vi "Framework Test.vi"() -> ()   [LabVIEW 2017]
uses:
  Typedefs/DSF Engine Framework Configuration.ctl
  Typedefs/DSF Engine Plugin Configuration.ctl
  Typedefs/DSF Timing Info.ctl
  Typedefs/DSF Engine Plugin Thread Configuration.ctl
  Typedefs/DSF Settings Info.ctl
  Typedefs/DSF Engine Transfer Group Configuration.ctl
  Typedefs/DSF Direction.ctl
  Typedefs/DSF Engine Transfer Configuration.ctl
  Typedefs/DSF Byte Order.ctl
  Typedefs/DSF Engine Channel Configuration.ctl
  Typedefs/DSF Data Type.ctl
  Typedefs/DSF Timeout Behavior.ctl
  Classes/Framework/Framework Options.ctl
  Typedefs/DSF FIFO Options.ctl
  Classes/Thread/Thread Options.ctl
  Typedefs/DSF Plugin Options.ctl
  Typedefs/DSF Performance Options.ctl
  Classes/Framework/Data Server Options.ctl
  <vilib>/NI/Memory Manager/Classes/Pointer/Pointer.lvclass/Pointer.ctl
  <vilib>/NI/Memory Manager/Classes/Pointer/Write Bool.vi
  <vilib>/NI/Memory Manager/Classes/Pointer/Write DBL.vi
  <vilib>/NI/Memory Manager/Classes/Pointer/Read Bool.vi
  <vilib>/NI/Memory Manager/Classes/Pointer/Set Address.vi
  <vilib>/NI/Memory Manager/Classes/Pointer/Set Size.vi
  <vilib>/NI/Memory Manager/Classes/Pointer/Set Internal.vi
  <vilib>/NI/Memory Manager/Classes/Pointer/Write (No Check).vi
  <vilib>/NI/Memory Manager/Classes/Pointer/Write (No Check) Bool.vi
  <vilib>/NI/Memory Manager/Classes/Pointer/Check Move.vi
  <vilib>/NI/Memory Manager/Classes/Pointer/Check Null Pointer.vi
  <vilib>/NI/Memory Manager/Classes/Pointer/Clear (No Check).vi
  <vilib>/NI/Memory Manager/Classes/Pointer/Check Length.vi
  <vilib>/NI/Memory Manager/Classes/Pointer/Write (No Check) DBL.vi
  <vilib>/NI/Memory Manager/Classes/Pointer/Read (No Check).vi
  <vilib>/NI/Memory Manager/Classes/Pointer/Read (No Check) Bool.vi
  <vilib>/NI/Memory Manager/Classes/Pointer/Get Internal.vi
  <vilib>/NI/Memory Manager/Classes/Pointer/Errors.vi
  <vilib>/NI/Memory Manager/Classes/Pointer/Zone.vi
  <vilib>/NI/Memory Manager/Classes/Pointer/Check Count.vi
  <vilib>/NI/Memory Manager/Classes/Pointer/Check Bounds (Power of 2).vi
  <vilib>/NI/Memory Manager/Classes/Pointer/Null Pointer.vi
  <vilib>/NI/Memory Manager/Classes/Pointer/Is Null.vi
  <vilib>/NI/Memory Manager/Classes/Pointer/Check Bounds (Pointer).vi
  <vilib>/NI/Memory Manager/Classes/Pointer/Create Error.vi
  <vilib>/NI/Memory Manager/Classes/Pointer/Out of Bounds.vi
  <vilib>/NI/Memory Manager/Classes/Pointer/Check Bounds.vi
  <vilib>/NI/Memory Manager/Constants/Constants.vi
  <vilib>/NI/Memory Manager/Constants/Library Name.vi
  <vilib>/NI/Memory Manager/Classes/Pointer/Pointer Error Info.vi
  <vilib>/NI/Memory Manager/Constants/Pointer Class Name.vi
  <vilib>/NI/Memory Manager/Classes/Pointer/Write Pointer Size to Error.vi
  <vilib>/NI/Memory Manager/Classes/Pointer/Check Bounds (Buffer).vi
  <vilib>/NI/Memory Manager/Classes/Pointer/Buffer Underflow.vi
  <vilib>/NI/Memory Manager/VIs/New Error Cluster.vi
  <vilib>/NI/Memory Manager/VIs/New Error Cluster (512B).vi
  <vilib>/NI/Memory Manager/VIs/Set Error Status.vi
  <vilib>/NI/Memory Manager/VIs/Set Error Code.vi
  <vilib>/NI/Memory Manager/VIs/Set Error Source.vi
  <vilib>/NI/Memory Manager/VIs/Write String to Source.vi
  <vilib>/NI/Memory Manager/VIs/Write Numeric to Source.vi
  <vilib>/NI/Memory Manager/VIs/Write Numeric Scalar to Source (Base10 U64).vi
  Classes/Configuration/Channel Count (Framework).vi
  <vilib>/NI/Memory Manager/Classes/Pointer/Pointer.lvclass
  Classes/Framework/Framework.lvclass
  Classes/Configuration/Configuration Session.lvclass
  DSF Core.lvlib
  Classes/Thread/Thread.lvclass
panel:
  in  "first channel":dbl format="%.3f"
  out "iteration":u64
  out "error out":errorcluster
  in  "framework options":T1={"FIFO Options"={"Infinite Timeouts"=FALSE}, "Thread Options"={"Show FP On Call"=TRUE, "Close FP After Call"=TRUE, "Allow Debugging"=TRUE}, "Plugin Options"={"Default Components"=TRUE}, "Performance Options"={"Measure Period"=TRUE, "Measure Rx/Tx Duration"=TRUE}, "Data Server Options"={"Enable Data Server"=TRUE, "Period"=50}} {"Data Server Options"."Period" format="%d ms"}
  in  "framework configuration":T7
  in  "stop":bool
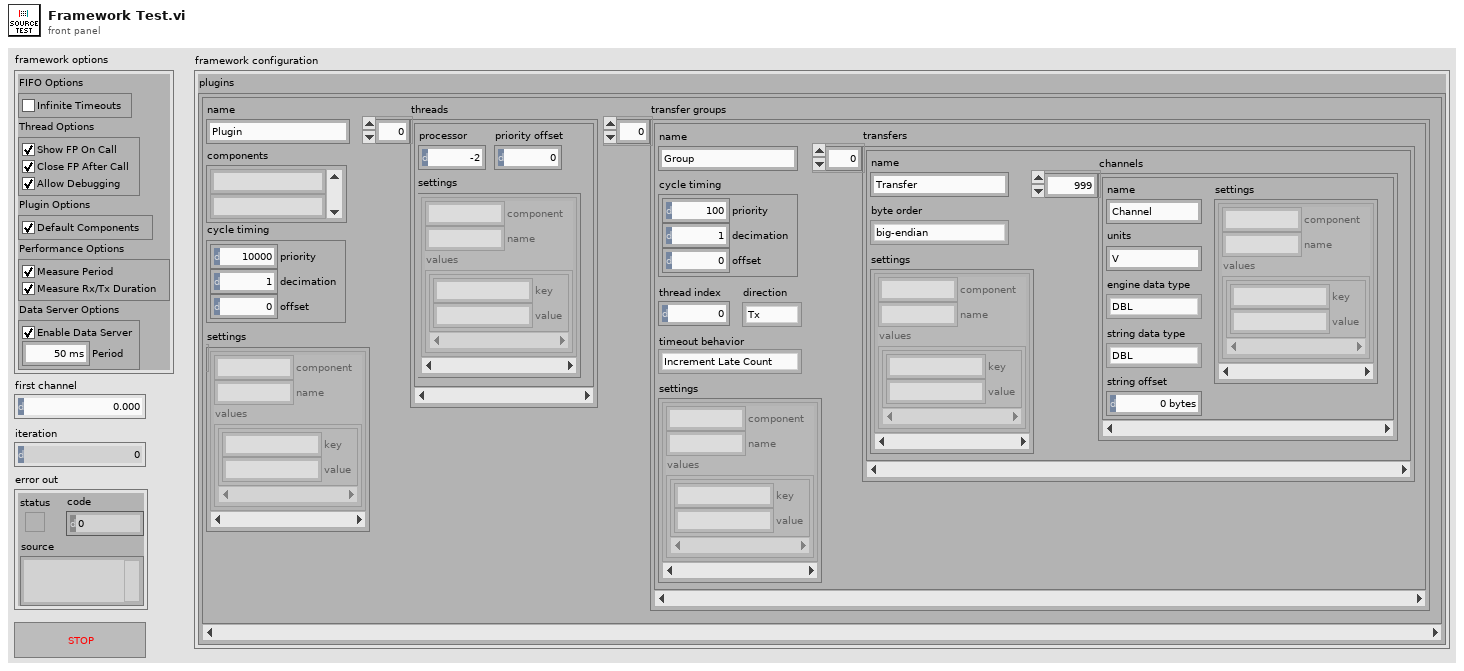
[diagram p1: front panel]
types:
  T1 = typedef "DSF Core.lvlib/Framework.lvclass/Framework Options.ctl" = cluster{"FIFO Options":T2, "Thread Options":T3, "Plugin Options":T4, "Performance Options":T5, "Data Server Options":T6}
  T2 = typedef "DSF Core.lvlib/Framework.lvclass/DSF FIFO Options.ctl" = cluster{"Infinite Timeouts":bool}
  T3 = typedef "DSF Core.lvlib/Thread.lvclass/Thread Options.ctl" = cluster{"Show FP On Call":bool, "Close FP After Call":bool, "Allow Debugging":bool}
  T4 = typedef "DSF Core.lvlib/Framework.lvclass/DSF Plugin Options.ctl" = cluster{"Default Components":bool}
  T5 = typedef "DSF Core.lvlib/DSF Performance Options.ctl" = cluster{"Measure Period":bool, "Measure Rx/Tx Duration":bool}
  T6 = typedef "DSF Core.lvlib/Framework.lvclass/Data Server Options.ctl" = cluster{"Enable Data Server":bool, "Period":u32}
  T7 = typedef "DSF Core.lvlib/DSF Engine Framework Configuration.ctl" = cluster{"plugins":T8[]}
  T8 = typedef "DSF Core.lvlib/DSF Engine Plugin Configuration.ctl" = cluster{"name":string, "components":string[], "cycle timing":T9, "threads":T10[], "transfer groups":T12[], "settings":T11}
  T9 = typedef "DSF Core.lvlib/DSF Timing Info.ctl" = cluster{"priority":u64, "decimation":u64, "offset":u64}
  T10 = typedef "DSF Core.lvlib/DSF Engine Plugin Thread Configuration.ctl" = cluster{"processor":i32, "priority offset":i16, "settings":T11}
  T11 = typedef "DSF Core.lvlib/DSF Settings Info.ctl" = cluster{"component":string, "name":string, "values":cluster{"key":string, "value":string}[]}[]
  T12 = typedef "DSF Core.lvlib/DSF Engine Transfer Group Configuration.ctl" = cluster{"name":string, "direction":T13, "cycle timing":T9, "thread index":i32, "settings":T11, "transfers":T14[], "timeout behavior":T18}
  T13 = typedef "DSF Core.lvlib/DSF Direction.ctl" = enum8{"Tx", "Rx"}
  T14 = typedef "DSF Core.lvlib/DSF Engine Transfer Configuration.ctl" = cluster{"name":string, "byte order":T15, "settings":T11, "channels":T16[]}
  T15 = typedef "DSF Core.lvlib/DSF Byte Order.ctl" = enum8{"big-endian", "little-endian"}
  T16 = typedef "DSF Core.lvlib/DSF Engine Channel Configuration.ctl" = cluster{"string offset":u64, "name":string, "units":string, "engine data type":T17, "string data type":T17, "settings":T11}
  T17 = typedef "DSF Core.lvlib/DSF Data Type.ctl" = enum8{"Bool", "SGL", "DBL", "I8", "I16", "I32", "I64", "U8", "U16", "U32", "U64"}
  T18 = typedef "DSF Core.lvlib/DSF Timeout Behavior.ctl" = enum8{"Increment Late Count", "Throw Error"}
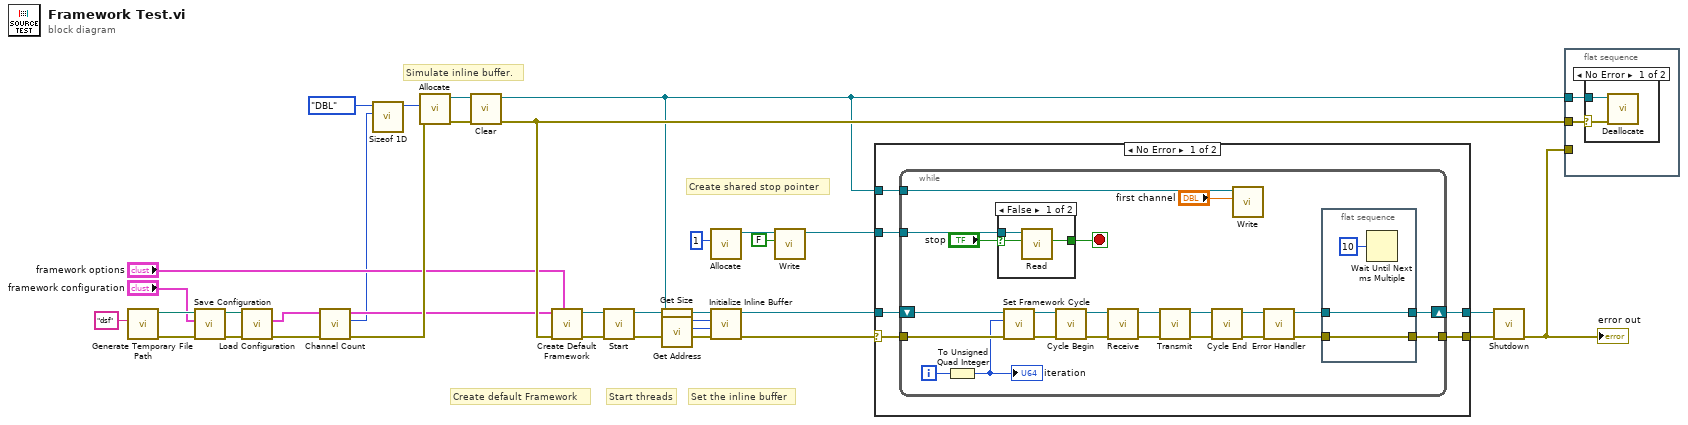
[diagram p0: block diagram]
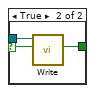
[diagram p3: hidden frame]
diagram:
  # "Create shared stop pointer"
  # "Set the inline buffer"
  # "Start threads"
  # "Create default Framework"
  # "Simulate inline buffer."
  n1 = call <vilib>:"Generate Temporary File Path.vi"("Temporary File Extension (tmp)"="dsf") -> ("error out"=w4:errorcluster, "Unique Temporary File Path"=w9:path)  [unwired: 9 in]
  n2 = call "Save Configuration.vi"("error in (no error)"=w4, "configuration"="framework configuration", "configuration file path"=w9) -> ("error out"=w6:errorcluster, "configuration file path dup"=w5:path)  [unwired: 5 in, 2 out]
  n3 = call "Load Configuration.vi"("error in (no error)"=w6, "configuration file path"=w5) -> ("error out"=w8:errorcluster, "configuration"=w7:T7)  [unwired: 6 in, 2 out]
  n4 = call-poly "Channel Count.vi"("error in (no error)"=w8, "Framework Configuration in"=w7) -> ("error out"=w13:errorcluster, "total channel count"=w1:u64, "Framework Configuration out"=w12:T7)  [unwired: 7 in]
  n5 = call "Sizeof 1D.vi"("count"=w1, "data type"=DSF_Data_Type."DBL") -> ("size in bytes"=w11:u64)  [unwired: 9 in]
  n6 = call <vilib>:"Allocate.vi"("error in (no error)"=w13, "size"=w11) -> ("error out"=w29:errorcluster, "Pointer out"=w26:refnum<class "Pointer.lvclass">)  [unwired: 8 in]
  n7 = call <vilib>:"Clear.vi"("error in (no error)"=w29, "Pointer in"=w26) -> ("error out"=w33:errorcluster, "Pointer out"=w15:refnum<class "Pointer.lvclass">)  [unwired: 8 in]
  n8 = call "Create Default Framework.vi"("framework options"="framework options", "error in (no error)"=w33, "framework configuration"=w12) -> ("error out"=w20:errorcluster, "Framework"=w25:refnum<class "Framework.lvclass">)  [unwired: 7 in]
  n9 = call-dynamic "Start.vi"("error in (no error)"=w20, "Framework in"=w25) -> ("error out"=w24:errorcluster, "Framework out"=w32:refnum<class "Framework.lvclass">)  [unwired: 8 in]
  n10 = call <vilib>:"Get Address.vi"("Pointer in"=w15) -> ("address"=w27:u64)  [unwired: 9 in, 1 out]
  n11 = call <vilib>:"Get Size.vi"("Pointer in"=w15) -> ("size"=w28:u64)  [unwired: 9 in, 1 out]
  n12 = call <vilib>:"Allocate.vi"("size"=u64 1) -> ("Pointer out"=w22:refnum<class "Pointer.lvclass">)  [unwired: 9 in, 1 out]
  n13 = call "Initialize Inline Buffer.vi"("error in (no error)"=w24, "size"=w28, "address"=w27, "Framework in"=w32) -> ("error out"=w18:errorcluster, "Framework out"=w16:refnum<class "Framework.lvclass">)  [unwired: 6 in]
  n14 = call-poly <vilib>:"Write.vi"("value"=FALSE, "Pointer in"=w22) -> ("Pointer out"=w17:refnum<class "Pointer.lvclass">)  [unwired: 6 in, 3 out]
  n15 = case shown="No Error" w18 {
    selector: w18 -> [w38 w72]
    tunnel: [w36 w72] -> w31
    tunnel: w16 -> [w39 w73]
    tunnel: [w37 w73] -> w30
    tunnel: w17 -> [w35 _]
    tunnel: w15 -> [w34 _]
    frame No Error {
      n16 = while {
        shift-right: [w60] -> w37
        shift-left: w39 -> [w54]
        tunnel: w35 -> [w57]
        tunnel: w38 -> [w53]
        tunnel: [w59] -> w36
        tunnel: w34 -> [w41]
        i -> [w58]
        stop <- w55 stop-if-true
        n17 = To Unsigned Quad Integer(1:w58) -> (0:w52:u64)
        "iteration" <- w52
        n18 = case shown="False" "stop" {
          selector: "stop" -> [w64 w67]
          tunnel: w57 -> [w65 w68]
          tunnel: [w63 w66] -> w55
          frame False {
            n19 = call-poly <vilib>:"Read.vi"("value in"=w64, "Pointer in"=w65) -> ("value out"=w63:bool)  [unwired: 6 in, 3 out]
          }
          frame True {
            n20 = call-poly <vilib>:"Write.vi"("value"=w67, "Pointer in"=w68) -> ("value"=w66:bool)  [unwired: 6 in, 3 out]
          }
        }
        n21 = call "Set Framework Cycle.vi"("error in (no error)"=w53, "iteration"=w52, "Framework in"=w54) -> ("error out"=w50:errorcluster, "Framework out"=w51:refnum<class "Framework.lvclass">)  [unwired: 7 in]
        n22 = call "Cycle Begin.vi"("error in (no error)"=w50, "Framework in"=w51) -> ("error out"=w48:errorcluster, "Framework out"=w49:refnum<class "Framework.lvclass">)  [unwired: 8 in]
        n23 = call "Receive.vi"("error in (no error)"=w48, "Framework in"=w49) -> ("error out"=w62:errorcluster, "Framework out"=w61:refnum<class "Framework.lvclass">)  [unwired: 8 in]
        n24 = call "Transmit.vi"("error in (no error)"=w62, "Framework in"=w61) -> ("error out"=w46:errorcluster, "Framework out"=w47:refnum<class "Framework.lvclass">)  [unwired: 8 in]
        n25 = call "Cycle End.vi"("error in (no error)"=w46, "Framework in"=w47) -> ("error out"=w44:errorcluster, "Framework out"=w45:refnum<class "Framework.lvclass">)  [unwired: 8 in]
        n26 = call-poly <vilib>:"Write.vi"("value"="first channel", "Pointer in"=w41) -> ()  [unwired: 6 in, 4 out]
        n27 = call "Error Handler.vi"("error in (no error)"=w44, "Framework in"=w45) -> ("error out"=w42:errorcluster, "Framework out"=w43:refnum<class "Framework.lvclass">)  [unwired: 8 in]
        n28 = flat-sequence {
          tunnel: w43 -> [w70]
          tunnel: w42 -> [w69]
          tunnel: [w70] -> w60
          tunnel: [w69] -> w59
          frame #0 {
            n29 = Wait Until Next ms Multiple(millisecond multiple=u32 10 ("milliseconds to wait")) -> ()  [unwired: 1 out]
          }
        }
      }
    }
    frame Error {
    }
  }
  n30 = call-dynamic "Shutdown.vi"("error in (no error)"=w31, "Framework in"=w30) -> ("error out"=w19:errorcluster)  [unwired: 8 in, 1 out]
  "error out" <- w19
  n31 = flat-sequence {
    tunnel: w15 -> [w75]
    tunnel: w19 -> [_]
    tunnel: w33 -> [w74]
    frame #0 {
      n32 = case shown="No Error" w74 {
        selector: w74 -> [w76 _]
        tunnel: w75 -> [w77 _]
        frame No Error {
          n33 = call <vilib>:"Deallocate.vi"("error in (no error)"=w76, "Pointer"=w77) -> ()  [unwired: 8 in, 2 out]
        }
        frame Error {
        }
      }
    }
  }
